vi "JL - Verify Display.vi"(0 "GEA2 Reference In":refnum<k24>, 1 "Model Select":T8, 5 "Expected LEDs":T1={"SSD"="", "Cycle Selection"=enum."Cycle 0", "Bar Selection"=enum."Bar 1", "Temp Setting"=enum."High", "Dryness Level"=enum."Extra Dry", "Time Setting"=enum."Default Time 5", "Dryer Status"=enum."Status 6", "Start/Pause"=FALSE, "Pause"=FALSE, "Control Lock"=FALSE, "Sensing"=FALSE, "Clean Filter"=FALSE, "My Cycle"=FALSE, "Delay Dry"=FALSE, "Volume"=FALSE, "Damp Alert"=FALSE, "Ext Tumble"=FALSE, "Decrement"=FALSE, "Increment"=FALSE, "eDry"=FALSE, "Extra Status"=FALSE}, 7 "Care?":T9, 11 "Error In":errorcluster) -> (4 "GEA2 Reference Out":refnum<k24>, 6 "Pass/Fail?":bool, 8 "Report Text":string, 15 "Error Out":errorcluster)   [LabVIEW 2016]
doc: "This VI is used to verify the display on the HEUI."
uses:
  Q:/Common/DLLs/GEA3/GeaCommunication.dll
  Common/DLLs/GEA3/GeaCommunication.dll
  type defs/JL Display Care.ctl
  type defs/JL Display.ctl
  type defs/Cycle Selection Enum.ctl
  type defs/Bar Enum.ctl
  type defs/Temp Setting Enum.ctl
  type defs/Dryness Enum.ctl
  type defs/Time Enum.ctl
  type defs/Status Enum.ctl
  type defs/JL_Trans-Model.ctl
  Common/LabVIEW GEA2 Toolkit/LabVIEW_GEA2_Toolkit.lvlibp/type defs/ERD Read Data In.ctl
  Common/LabVIEW GEA2 Toolkit/LabVIEW_GEA2_Toolkit.lvlibp/type defs/Data Type.ctl
  Common/LabVIEW GEA2 Toolkit/LabVIEW_GEA2_Toolkit.lvlibp/type defs/Source_Destination.ctl
  Common/LabVIEW GEA2 Toolkit/LabVIEW_GEA2_Toolkit.lvlibp
panel:
  out "Actual LEDs":T1={"SSD"="", "Cycle Selection"=enum."Cycle 0", "Bar Selection"=enum."Bar 1", "Temp Setting"=enum."High", "Dryness Level"=enum."Extra Dry", "Time Setting"=enum."Default Time 5", "Dryer Status"=enum."Status 6", "Start/Pause"=FALSE, "Pause"=FALSE, "Control Lock"=FALSE, "Sensing"=FALSE, "Clean Filter"=FALSE, "My Cycle"=FALSE, "Delay Dry"=FALSE, "Volume"=FALSE, "Damp Alert"=FALSE, "Ext Tumble"=FALSE, "Decrement"=FALSE, "Increment"=FALSE, "eDry"=FALSE, "Extra Status"=FALSE}
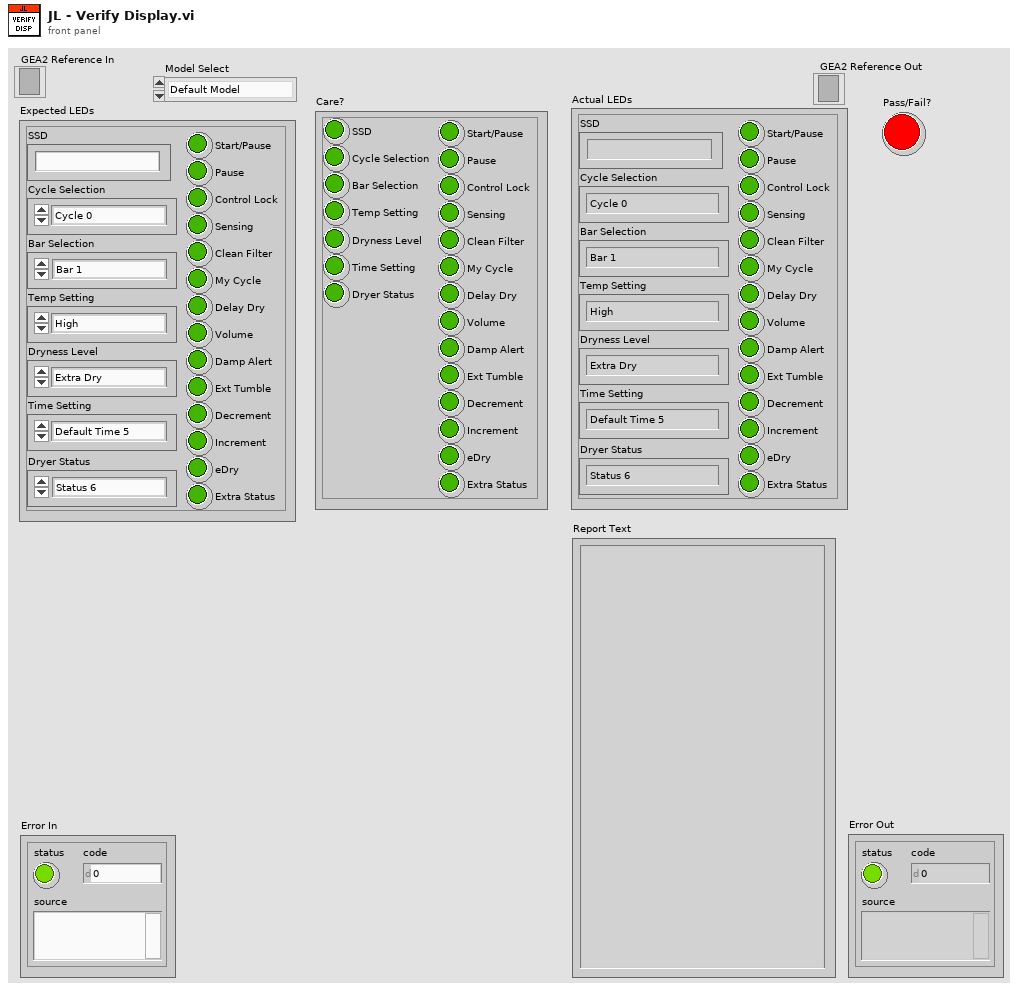
[diagram p1: front panel]
types:
  T1 = typedef "JL Display.ctl" = cluster{"SSD":string, "Cycle Selection":T2, "Bar Selection":T3, "Temp Setting":T4, "Dryness Level":T5, "Time Setting":T6, "Dryer Status":T7, "Start/Pause":bool, "Pause":bool, "Control Lock":bool, "Sensing":bool, "Clean Filter":bool, "My Cycle":bool, "Delay Dry":bool, "Volume":bool, "Damp Alert":bool, "Ext Tumble":bool, "Decrement":bool, "Increment":bool, "eDry":bool, "Extra Status":bool}
  T2 = typedef "Cycle Selection Enum.ctl" = enum16{"Cycle 0", "Cycle 1", "Cycle 2", "Cycle 3", "Cycle 4", "Cycle 5", "Cycle 6", "Cycle 7", "Cycle 8", "Cycle 9", "Cycle 10", "Cycle 11", "Cycle 12", "Cycle 13", "Off", "*Invalid"}
  T3 = typedef "Bar Enum.ctl" = enum16{"Bar 1", "Bar 2", "Bar 3", "Bar 4", "Bar 5", "Off", "*Incorrect*"}
  T4 = typedef "Temp Setting Enum.ctl" = enum16{"Off", "No Heat", "Extra Low", "Low", "Medium", "High", "*Incorrect*"}
  T5 = typedef "Dryness Enum.ctl" = enum16{"Off", "Damp", "Less Dry", "Dry", "More Dry", "Extra Dry", "*Incorrect*"}
  T6 = typedef "Time Enum.ctl" = enum16{"Off", "Default Time 1", "Default Time 2", "Default Time 3", "Default Time 4", "Default Time 5", "*Incorrect*"}
  T7 = typedef "Status Enum.ctl" = enum16{"Status 1", "Status 2", "Status 3", "Status 4", "Status 5", "Status 6", "Off", "*Incorrect*"}
  T8 = typedef "JL_Trans-Model.ctl" = enum16{"Default Model"}
  T9 = typedef "JL Display Care.ctl" = cluster{"SSD":bool, "Cycle Selection":bool, "Bar Selection":bool, "Temp Setting":bool, "Dryness Level":bool, "Time Setting":bool, "Dryer Status":bool, "Start/Pause":bool, "Pause":bool, "Control Lock":bool, "Sensing":bool, "Clean Filter":bool, "My Cycle":bool, "Delay Dry":bool, "Volume":bool, "Damp Alert":bool, "Ext Tumble":bool, "Decrement":bool, "Increment":bool, "eDry":bool, "Extra Status":bool}
  T10 = typedef "LabVIEW_GEA2_Toolkit.lvlibp/Source_Destination.ctl" = cluster{"Source":u8, "Destination":u8}
  T11 = typedef "LabVIEW_GEA2_Toolkit.lvlibp/ERD Read Data In.ctl" = cluster{"ERD Number":u16, "Data Type":T12}
  T12 = typedef "LabVIEW_GEA2_Toolkit.lvlibp/Data Type.ctl" = enum16{"string", "boolean", "uint8_t", "uint16_t", "uint32_t", "uint64_t", "int8_t", "int16_t", "int32_t", "int64_t"}
  T13 = typedef "LabVIEW_GEA2_Toolkit.lvlibp/ERD Read Data Out.ctl" = cluster{"ERD Number":u16, "Data":string}
  T14 = typedef "UI_LEDs.ctl" = cluster{"Z301 - Encoder 0":bool, "Z302 - Encoder 13":bool, "Z303 - Encoder 12":bool, "Z304 - Encoder 11":bool, "Z305 - Encoder 10":bool, "Z306 - Encoder 09":bool, "Z307 - Encoder 08":bool, "Z308 - Encoder 07":bool, "Z309 - Encoder 06":bool, "Z310 - Encoder 05":bool, "Z311 - Encoder 04":bool, "Z312 - Encoder 03":bool, "Z313 - Encoder 02":bool, "Z314 - Encoder 01":bool, "Z315 - Unpopulated":bool, "Z316 - Unpopulated":bool, "Z317 - SSD1:A":bool, "Z318 - SSD1:B":bool, "Z319 - SSD1:G":bool, "Z320 - SSD1:C":bool, "Z321 - SSD1:D":bool, "Z322 - SSD1:E":bool, "Z323 - SSD1:F":bool, "Z324 - Pause 1":bool, "Z325 - Control Lock 1":bool, "Z326 - Sensing 1":bool, "Z327 - Clean Lint Filter 1":bool, "Z328 - Extra Status 1":bool, "Z329 - Extra Status 2":bool, "Z330 - Clean Lint Filter 2":bool, "Z331 -Sensing 2":bool, "Z332 - Unpopulated":bool, "Z333 - SSD2:A":bool, "Z334 - SSD2:B":bool, "Z335 - SSD2:G":bool, "Z345 - SSD2:C":bool, "Z336 - SSD2:D":bool, "Z337 - SSD2:E":bool, "Z338 - SSD2:F":bool, "Z339 - Pause 3":bool, "Z340 - Control Lock 3":bool, "Z353 - Sensing 3":bool, "Z342 - Clean Lint Filter 3":bool, "Z344 - Extra Status 3":bool, "Z346 - Extra Status 4":bool, "Z341 - Pause 2":bool, "Z343 - Control Lock 2":bool, "Z347 - Unpopulated":bool, "Z348 -My Cycle":bool, "Z349 - Delay Dry":bool, "Z350 - Volume":bool, "Z351 - Damp Alert":bool, "Z352 - Bar 1":bool, "Z354 - Bar 2":bool, "Z355 - Bar 3":bool, "Z356 - Bar 4":bool, "Z357 - Bar 5":bool, "Z358 - eDry":bool, "Z359 - Time Increment":bool, "Z360 - Time Decrement":bool, "Z361 - Extended Tumble":bool, "Z362 - Unpopulated":bool, "Z363 - Unpopulated":bool, "Z364 - Unpopulated":bool, "Z365 - Status 1":bool, "Z366 - Status 3":bool, "Z367 - Default Time 5":bool, "Z368 - Default Time 4":bool, "Z369 - Default Time 3":bool, "Z370 - Dry":bool, "Z371 - Status 2":bool, "Z372 -Default Time 2":bool, "Z373 - Default Time 1":bool, "Z374 - Unpopulated":bool, "Z375 - Default Time 0":bool, "Z376 - No Heat":bool, "Z377 - Unpopulated":bool, "Z378 - Unpopulated":bool, "Z379 - Unpopulated":bool, "Z380 - Unpopulated":bool, "Z381 - Status 4":bool, "Z382 - Status 6":bool, "Z383 - More Dry":bool, "Z384 - High":bool, "Z385 - Medium":bool, "Z386 -Low":bool, "Z387 - Status 5":bool, "Z388 - Less Dry":bool, "Z388 - Extra Low":bool, "Z390 - Unpopulated":bool, "Z391 - Damp":bool, "Z392 - Unpopulated":bool, "Z393 - Unpopulated":bool, "Z394 - Unpopulated":bool, "Z395 - Unpopulated":bool, "Z396 - Unpopulated":bool, "Z101 - unpop?":bool, "Z102 - Start/Pause":bool, "OFF - OFF":bool, "MAX - MAX":bool}
  T15 = typedef "SB_LEDs.ctl" = cluster{"Z101 - Start/Pause":bool, "Z - unpop?":bool, "Z103 - Encoder 0":bool, "Z104 - Encoder 13":bool, "Z105 - Encoder 12":bool, "Z106 - Encoder 11":bool, "Z107 - Encoder 10":bool, "Z108 - Encoder 09":bool, "Z109 - Encoder 08":bool, "Z110 - Encoder 07":bool, "Z111 - Encoder 06":bool, "Z112 - Encoder 05":bool, "Z113 - Encoder 04":bool, "Z114 - Encoder 03":bool, "Z115 - Encoder 02":bool, "Z116 - Encoder 01":bool, "Z117 - Bar 1":bool, "Z118 - Bar 2":bool, "Z119 - Bar 3":bool, "Z120 - Bar 4":bool, "Z121 - Bar 5":bool, "Z122 - SSD1:A":bool, "Z123 - SSD1:B":bool, "Z124 - SSD1:C":bool, "Z125 - SSD1:D":bool, "Z126 - SSD1:E":bool, "Z127 - SSD1:F":bool, "Z128 - SSD1:G":bool, "Z129 - SSD2:A":bool, "Z130 - SSD2:B":bool, "Z131 - SSD2:C":bool, "Z132 - SSD2:D":bool, "Z133 - SSD2:E":bool, "Z134 - SSD2:F":bool, "Z135 - SSD2:G":bool, "Z136 - Pause 2":bool, "Z137 - Pause 3":bool, "Z138 - Control Lock 1":bool, "Z139 - Control Lock 2":bool, "Z140 - Control Lock 3":bool, "Z142 - Sensing 1":bool, "Z142 -Sensing 2":bool, "Z143 - Sensing 3":bool, "Z144 - Extra Status 1":bool, "Z145 - Extra Status 2":bool, "Z146 - Extra Status 3":bool, "Z147 - Extra Status 4":bool, "Z148 - Status 1":bool, "Z149 - Status 2":bool, "Z150 - Status 3":bool, "Z151 - Status 4":bool, "Z152 - Status 5":bool, "Z153 - Status 6":bool, "Z154 - Default Time 5":bool, "Z155 - Default Time 4":bool, "Z153 - Default Time 3":bool, "Z157 -Default Time 2":bool, "Z158 - Default Time 1":bool, "Z159 - Default Time 0":bool, "Z160 - More Dry":bool, "Z161 - Dry":bool, "Z162 - Less Dry":bool, "Z163 - Damp":bool, "Z164 - High":bool, "Z165 - Medium":bool, "Z166 - Extra Low":bool, "Z167 - No Heat":bool, "Z168 - Volume":bool, "Z169 - Damp Alert":bool, "Z170 - Extended Tumble":bool, "Z171 - Time Decrement":bool, "Z172 - Time Increment":bool, "Z173 - eDry":bool, "Z174 -My Cycle":bool, "Z175 - Delay Dry":bool, "Z176 - Clean Lint Filter 1":bool, "Z177 - Clean Lint Filter 2":bool, "Z178 - Clean Lint Filter 3":bool, "Z179 - Pause 1":bool, "OFF - OFF":bool, "MAX - MAX":bool, "Z165B -Low":bool}
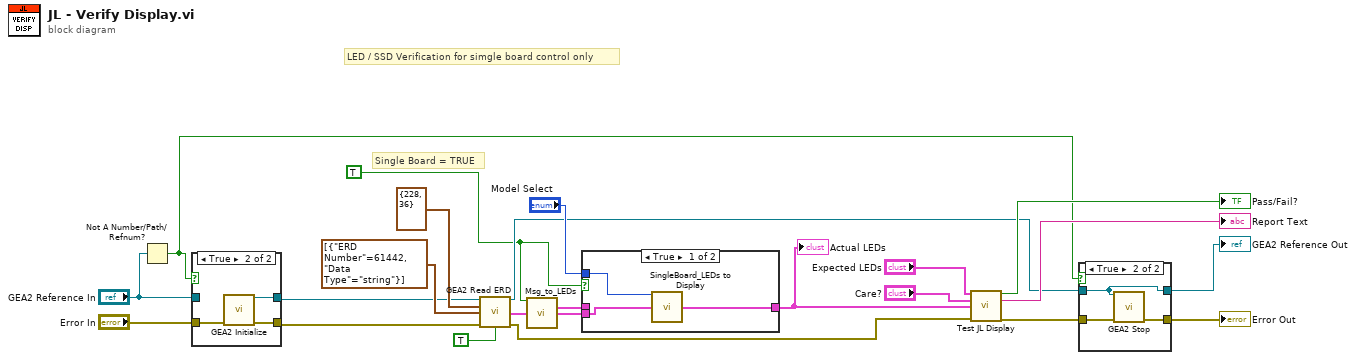
[diagram p0: block diagram]
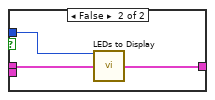
[diagram p3: hidden frame]
diagram:
  w3 = TRUE ("Verify ERD Response?")
  # "LED / SSD Verification for simgle board control only"
  # "Single Board = TRUE"
  n1 = Not A Number/Path/Refnum?(number/path/refnum="GEA2 Reference In") -> (NaN/Path/Refnum?=w4:bool)
  n2 = case shown="True" w4 {
    tunnel: [w24 w28] -> w2
    tunnel: "Error In" -> [w24 w27]
    tunnel: [w25 w26] -> w1
    tunnel: "GEA2 Reference In" -> [w25 _]
    frame False {
    }
    frame True {
      n3 = call "GEA2 Initialize.vi"("error in"=w27) -> ("GEA2 Reference Out"=w26:refnum<k24>, "error out"=w28:errorcluster)  [unwired: 12 in, 1 out]
    }
  }
  n4 = call "GEA2 Read ERD.vi"("GEA2 Reference In"=w1, "GEA Inputs"=T10 {"Source"=228, "Destination"=36}, "Read ERD List"=T11[] [{"ERD Number"=61442, "Data Type"=enum."string"}], "Error In"=w2, "Verify ERD Response?"=TRUE) -> ("GEA2 Reference Out"=w8:refnum<k24>, "ERD Data Out"=w19:T13[], "Error Out"=w5:errorcluster)  [unwired: 7 in, 1 out]
  n5 = call "Msg_to_LEDs.vi"("SingleBoard?"=w3, "ERD Data Out"=w19) -> ("Justice League UI"=w17:T14, "Justice League SB"=w11:T15)  [unwired: 10 in, 2 out]
  n6 = case shown="True" w3 {
    tunnel: w17 -> [_ w34]
    tunnel: "Model Select" -> [w31 w33]
    tunnel: w11 -> [w30 _]
    tunnel: [w29 w32] -> w10
    frame True {
      n7 = call "SingleBoard_LEDs to Display.vi"("Model Select"=w31, "Justice League SingleBoard Map"=w30) -> ("JL Display"=w29:T1)  [unwired: 13 in]
    }
    frame False {
      n8 = call "LEDs to Display.vi"("Model Select"=w33, "Justice League UI"=w34) -> ("JL Display"=w32:T1)  [unwired: 13 in]
    }
  }
  "Actual LEDs" <- w10
  n9 = call "Test JL Display.vi"("Expected LEDs"="Expected LEDs", "Care?"="Care?", "Actual LEDs"=w10, "error in"=w5) -> ("Pass/Fail?"=→"Pass/Fail?":bool, "Report Text"=→"Report Text":string, "error out"=w9:errorcluster)  [unwired: 9 in]
  n10 = case shown="True" w4 {
    tunnel: w9 -> [w35 w39]
    tunnel: [w35 w38] -> w6
    tunnel: [w36 w37] -> w7
    tunnel: w8 -> [w36 w37]
    frame False {
    }
    frame True {
      n11 = call "GEA2 Stop.vi"("GEA2 Reference In"=w37, "Error In"=w39) -> ("Error Out"=w38:errorcluster)  [unwired: 13 in]
    }
  }
  "GEA2 Reference Out" <- w7
  "Error Out" <- w6
